vi "dT.vi"(8 "error in (no error)":errorcluster, 11 "PID in":refnum<class "PID.lvclass">) -> (0 "error out":errorcluster, 2 "dT":dbl, 3 "PID out":refnum<class "PID.lvclass">)   [LabVIEW 2020, in "IG PID.lvlib" / "PID.lvclass"]
uses:
  PID.lvclass
  PID.lvclass/PID.ctl
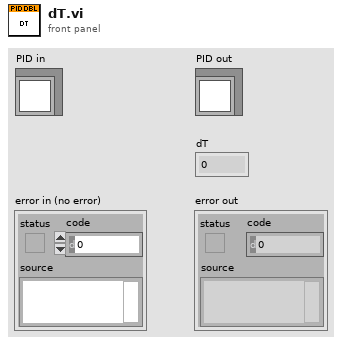
[diagram p1: front panel]
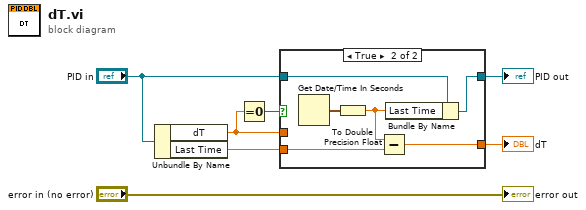
[diagram p0: block diagram]
diagram:
  n1 = Unbundle By Name("PID in") -> ("dT"=w5:dbl, "Last Time"=w4:dbl)
  n2 = Equal To 0?(x=w5) -> (x = 0?=w6:bool)
  n3 = case shown="True" w6 {
    tunnel: w5 -> [w9 _]
    tunnel: w4 -> [_ w14]
    tunnel: [w9 w13] -> w3
    tunnel: "PID in" -> [w8 w12]
    tunnel: [w8 w10] -> w1
    frame False {
    }
    frame True {
      n4 = Get Date/Time In Seconds() -> (seconds since 1Jan1904=w15:timestamp)
      n5 = To Double Precision Float(number=w15) -> (double precision float=w11:dbl)
      n6 = Subtract(x=w11, y=w14) -> (x-y=w13:dbl)
      n7 = Bundle By Name(cluster=w12, "Last Time"=w11) -> (w10:refnum<class "PID.lvclass">)
    }
  }
  "PID out" <- w1
  "dT" <- w3
  "error out" <- "error in (no error)"
